vi "Practica 9 - Convertidor Binario-Numerico.vi"() -> ()   [LabVIEW 2023]
uses:
  <vilib>/express/express shared/transition.llb/Dynamic To Waveform Array.vi
  <vilib>/express/express arith-compare/Formula/Block/exnFormulaBlock how many pts in the wave.vi
  <vilib>/express/express shared/ex_Modify Signal Name.vi
  <vilib>/express/express shared/transition.llb/Waveform Array To Dynamic.vi
  <vilib>/express/express arith-compare/Formula/XNode/ExpressFormulaBlockNode.xnode
panel:
  in  "Peso 4":bool
  in  "Peso 3":bool
  in  "Peso 2":bool
  in  "Peso 1":bool
  out "Salida 2":dbl
  out "luz 3":bool
  out "luz 4":bool
  out "luz 2":bool
  out "Luz1":bool
  out "Salida":dbl
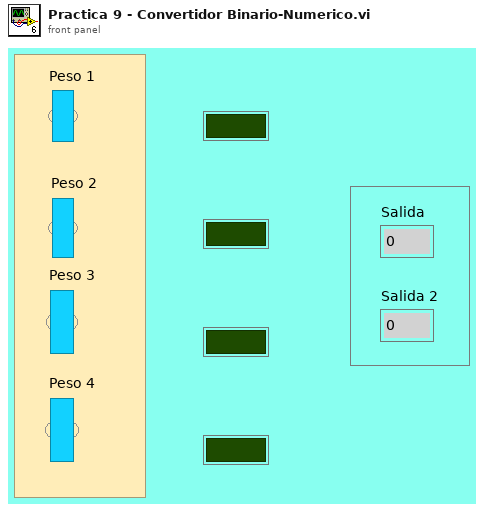
[diagram p1: front panel]
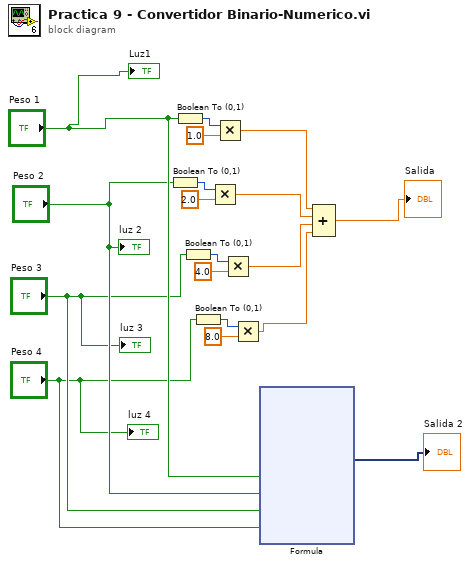
[diagram p0: block diagram]
diagram:
  n1 = Boolean To (0,1)(Boolean="Peso 2") -> (0, 1=w15:i16)
  n2 = Boolean To (0,1)(Boolean="Peso 1") -> (0, 1=w17:i16)
  n3 = Boolean To (0,1)(Boolean="Peso 3") -> (0, 1=w13:i16)
  n4 = Boolean To (0,1)(Boolean="Peso 4") -> (0, 1=w11:i16)
  n5 = Multiply(x=w15, y=2.0) -> (x*y=w8:dbl)
  n6 = Multiply(x=w17, y=1.0) -> (x*y=w9:dbl)
  n7 = Multiply(x=w13, y=4.0) -> (x*y=w7:dbl)
  n8 = Multiply(x=w11, y=8.0) -> (x*y=w6:dbl)
  n9 = xnode "Formula"("X1"="Peso 1", "X2"="Peso 2", "X3"="Peso 3", "X4"="Peso 4") -> ("Result"=→"Salida 2":dynamicdata)  [unwired: 1 in, 1 out]
  n10 = Compound Arithmetic op=ADD(w9, w8, w7, w6) -> (→"Salida":dbl)
  "Luz1" <- "Peso 1"
  "luz 2" <- "Peso 2"
  "luz 4" <- "Peso 4"
  "luz 3" <- "Peso 3"
